vi "Drive Command Helper.vi"(7 "Description":string, 8 "Command Info In":T3, 11 "SubSystem Data":T1) -> (0 "Command Info Out":T3, 1 "Command Timing":cluster{"Start Time (ms)":u32, "Iterations":i32}, 3 "SubSystem Data":T1)   [LabVIEW 2020]
doc: "Commands use this VI to asynchronously notify the subsystem controller that a new command has been issued. It also deteremines whether to abort the existing command."
uses:
  Drive Setpoints.ctl
  Drive Operations.ctl
  <vilib>/Rock Robotics/WPI/Framework/Command Status Info.ctl
  <vilib>/Rock Robotics/WPI/Framework/Completion Status.ctl
  <vilib>/Rock Robotics/WPI/Framework/Completion Notifier.ctl
  Drive Published Globals.vi
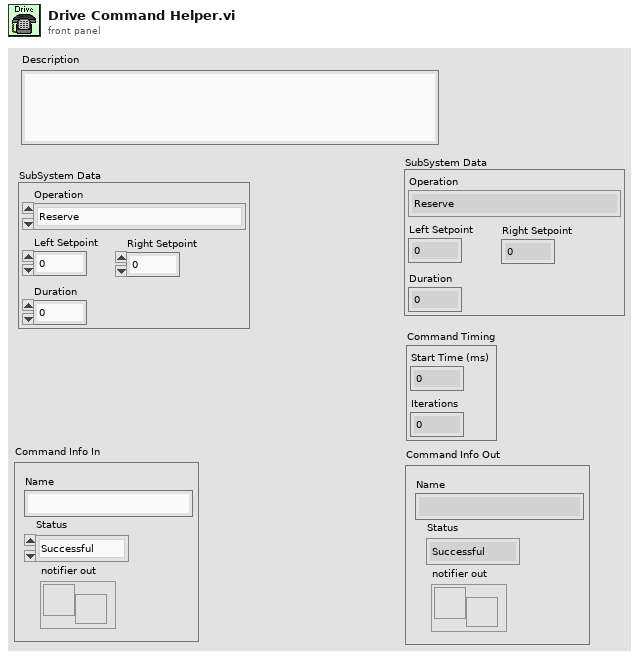
[diagram p1: front panel]
types:
  T1 = typedef "Drive Setpoints.ctl" = cluster{"Operation":T2, "Left Setpoint":dbl, "Right Setpoint":dbl, "Duration":dbl}
  T2 = typedef "Drive Operations.ctl" = enum16{"Reserve", "Read Current", "Immediate", "Drive for Time", "Drive for Distance", "Stop"}
  T3 = typedef "Command Status Info.ctl" = cluster{"Name":string, "Status":T4, "notifier out":T5}
  T4 = typedef "Completion Status.ctl" = enum16{"Successful", "Aborted", "Incomplete"}
  T5 = typedef "Completion Notifier.ctl" = refnum<notifier>
  T6 = cluster{"SubSystem Data":T1, cluster{"Start Time (ms)":u32, "Iterations":i32}, cluster{"Command Info":T3, "Description":string, "SubSystem Data":T1, "queue out":refnum<queue>, "Subsystem Name":string}}
  T7 = cluster{"SubSystem Data":T1, "Command Info In":T3, string}
  T8 = cluster{"Command Info":T3, "Description":string, "SubSystem Data":T1, "queue out":refnum<queue>, "Subsystem Name":string}
  T9 = cluster{"SubSystem Data":T1, "Command Info In":T3, "Description":string}
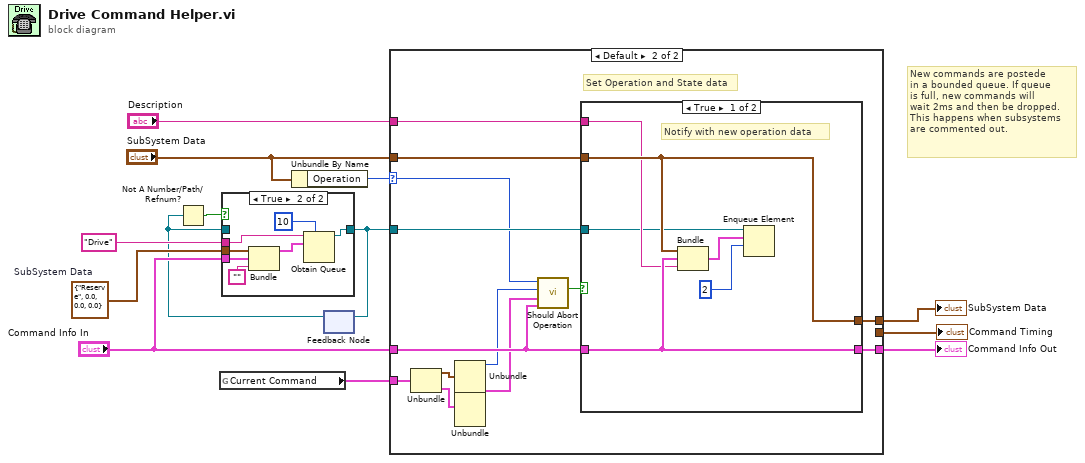
[diagram p0: block diagram]
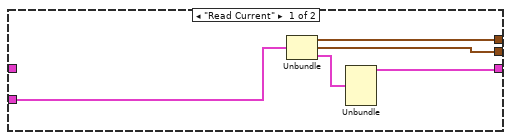
[diagram p3: hidden frame]
diagram:
  w7 = T1 {"Operation"=enum."Reserve", "Left Setpoint"=0.0, "Right Setpoint"=0.0, "Duration"=0.0}  # SubSystem Data
  # "New commands are postede\nin a bounded queue. If queue\nis full, new commands will\nwait 2ms and then be dropped.\nThis happens when subsystems\nare commented out."
  n1 = global read "Drive Published Globals.vi" "Current Command"() -> (w1:T6)
  n2 = Unbundle By Name("SubSystem Data") -> ("Operation"=w12:T2)
  n3 = feedback #1() -> (w4:refnum<queue>)  [unwired: 1 in]
  n4 = Not A Number/Path/Refnum?(number/path/refnum=w4) -> (NaN/Path/Refnum?=w5:bool)
  n5 = case shown="True" w5 {
    tunnel: "Drive" -> [_ w17]
    tunnel: [w14 w18] -> w10
    tunnel: w7 -> [_ w21]
    tunnel: "Command Info In" -> [_ w20]
    tunnel: w4 -> [w14 _]
    frame False {
    }
    frame True {
      n6 = Bundle("SubSystem Data"=w21, "Command Info In"=w20, "") -> (w16:T7)  [unwired: 1 in]
      n7 = Obtain Queue(max queue size (-1, unlimited)=10, name (unnamed)=w17, element data type=w16) -> (queue out=w18:refnum<queue>)  [unwired: 2 in, 2 out]
    }
  }
  n8 = feedback-in #1(w10) -> ()
  n9 = case shown="Default" w12 {
    selector: w12 -> [_ w34]
    tunnel: [w24 w36] -> w6
    tunnel: w10 -> [_ w38]
    tunnel: "SubSystem Data" -> [_ w39]
    tunnel: [w25 w37] -> w9
    tunnel: "Command Info In" -> [_ w33]
    tunnel: "Description" -> [_ w32]
    tunnel: [w23 _] -> w2
    tunnel: w1 -> [w22 w29]
    frame "Read Current" {
      n10 = Unbundle(w22) -> ("SubSystem Data"=w24:T1, w23:cluster{"Start Time (ms)":u32, "Iterations":i32}, w26:T8)
      n11 = Unbundle(w26) -> ("Command Info"=w25:T3)  [unwired: 4 out]
    }
    frame Default {
      # "Set Operation and State data"
      n12 = Unbundle(w29) -> ("SubSystem Data"=w30:T1, w31:T8)  [unwired: 1 out]
      n13 = Unbundle(w30) -> ("Operation"=w27:T2)  [unwired: 3 out]
      n14 = Unbundle(w31) -> ("Command Info"=w28:T3)  [unwired: 4 out]
      n15 = call <vilib>:"Should Abort Operation.vi"("New Command Info"=w33, "Command Info"=w28, "Current Operation"=w27, "New Operation"=w34) -> ("Execute"=w35:bool)  [unwired: 7 in]
      n16 = case shown="True" w35 {
        tunnel: [w45 w46] -> w36
        tunnel: w39 -> [w45 w46]
        tunnel: w38 -> [w42 _]
        tunnel: [w44 w47] -> w37
        tunnel: w33 -> [w44 w47]
        tunnel: w32 -> [w43 _]
        frame True {
          # "Notify with new operation data"
          n17 = Bundle("SubSystem Data"=w45, "Command Info In"=w44, "Description"=w43) -> (w41:T9)  [unwired: 1 in]
          n18 = Enqueue Element(queue=w42, element=w41, timeout in ms (-1)=2) -> ()  [unwired: 1 in, 3 out]
        }
        frame False {
          # "This operation will not be executed.\nUpstream command was aborted."
        }
      }
    }
  }
  "Command Info Out" <- w9
  "SubSystem Data" <- w6
  "Command Timing" <- w2
